vi "Task2.vi"() -> ()   [LabVIEW 2015]
uses:
  Global 15.vi
  Global 17.vi
  Global 12.vi
panel:
  out "String":string
  in  "stop":bool
  out "Sine 2":dynamicdata(graph) caption="Sine"
  out "Sine":dynamicdata(graph)
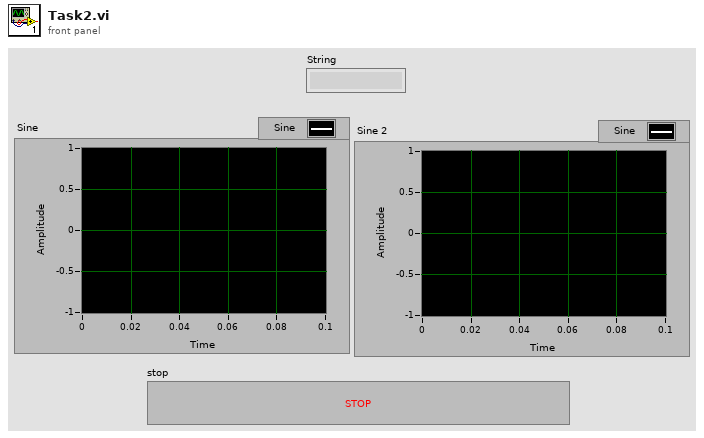
[diagram p1: front panel]
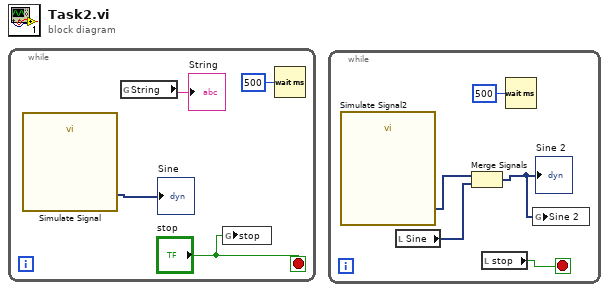
[diagram p0: block diagram]
diagram:
  n1 = while {
    stop <- "stop" stop-if-true
    n2 = call "Simulate Signal"() -> ("Sine"=→"Sine":dynamicdata)  [unwired: 14 in, 1 out]
    n3 = global read "Global 17.vi" "String"() -> (→"String":string)
    n4 = global write "Global 15.vi" "stop"("stop") -> ()
    n5 = Wait (ms)(milliseconds to wait=u32 500) -> ()  [unwired: 1 out]
  }
  n6 = while {
    stop <- w6 stop-if-true
    n7 = call "Simulate Signal2"() -> ("Sine"=w9:dynamicdata)  [unwired: 14 in, 1 out]
    n8 = local read "Sine"() -> (w7:dynamicdata)
    n9 = Merge Signals(w9, w7) -> (w5:dynamicdata)
    "Sine 2" <- w5
    n10 = local read "stop"() -> (w6:bool)
    n11 = Wait (ms)(milliseconds to wait=u32 500) -> ()  [unwired: 1 out]
    n12 = global write "Global 12.vi" "Sine 2"(w5) -> ()
  }
